vi "Spectrum Recorder.vi"() -> ()   [LabVIEW 2016]
uses:
  Libraries/Spectrum Recorder/Spectrum Recorder Configuration.ctl
  Libraries/Spectrum Recorder/Spectrum Recorder.lvclass
  Libraries/Spectrum Recorder/Spectrum Recorder.lvclass/Spectrum Recorder.ctl
  Libraries/Spectrum Recorder/Write Data file path indicator ref.vi
  Libraries/Spectrum Recorder/Write State ref.vi
  Libraries/Spectrum Recorder/Write Spectrum graph ref.vi
  <vilib>/ErrorRing/Error Ring.xnode
panel:
  in  "Open digitizer":bool
  out "State":bool
  out "Data file path":path=path "C:/Data"
  in  "Exit":bool
  in  "Stop":bool
  in  "Record":bool
  in  "Configuration":T1={"Start"=500000.0, "End"=2000000.0, "Duration"=40.0, "Filter time constant"=0.004, "Repeat (-1: forever)"=1, "Update rate"=1.0, "Data storage folder"=path "C:/Data"} {"Update rate" min=0.001 max=10.0 step=0.001 format="%#_6ps"; "Repeat (-1: forever)" format="%.0p"; "Filter time constant" format="%#_6ps"; "Duration" format="%#_6ps"; "End" format="%#_6pHz"; "Start" format="%#_6pHz"}
  out "Spectrum plot":cluster{dbl[], dbl[]}[](graph)
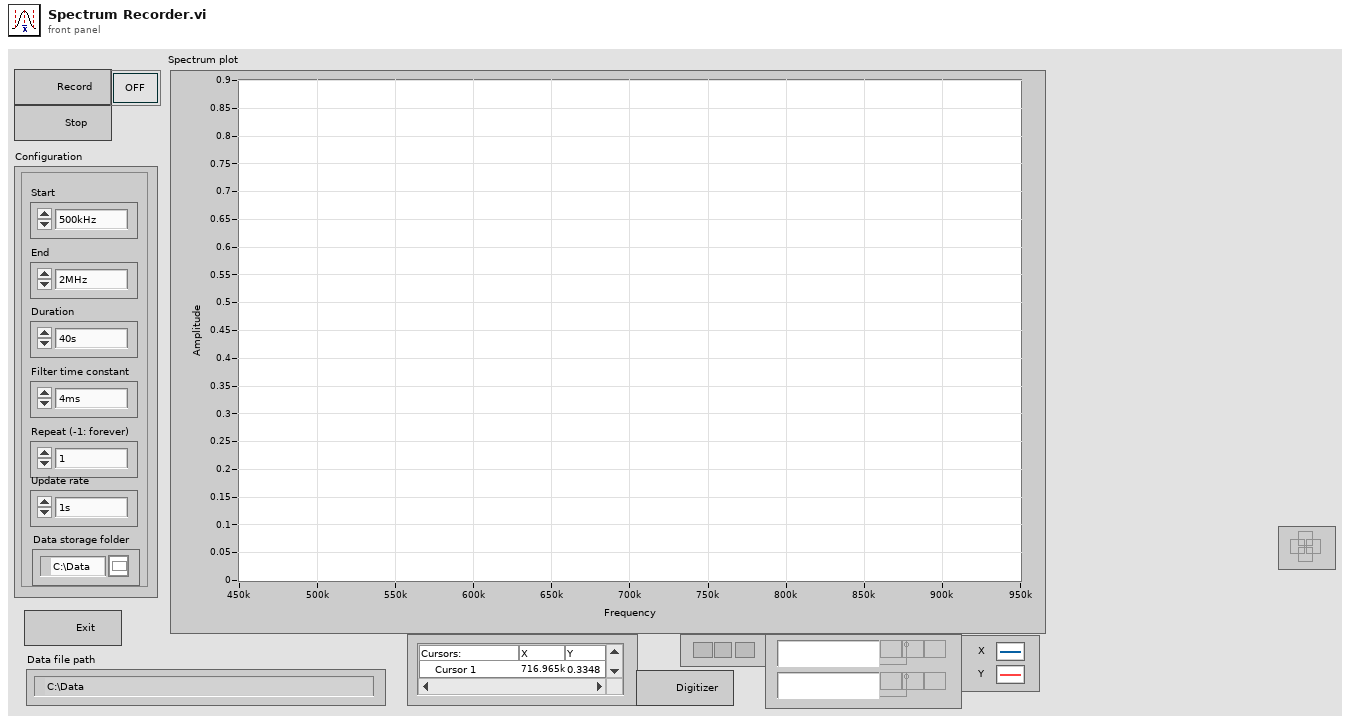
[diagram p1: front panel]
types:
  T1 = typedef "Spectrum Recorder Configuration.ctl" = cluster{"Start":dbl, "End":dbl, "Duration":dbl, "Filter time constant":dbl, "Repeat (-1: forever)":i32, "Update rate":dbl, "Data storage folder":path}
  T2 = enum32{"invalid app kind", "Development System", "Run Time System", "Student Edition", "Embedded LabVIEW", "Evaluation", "Custom"}
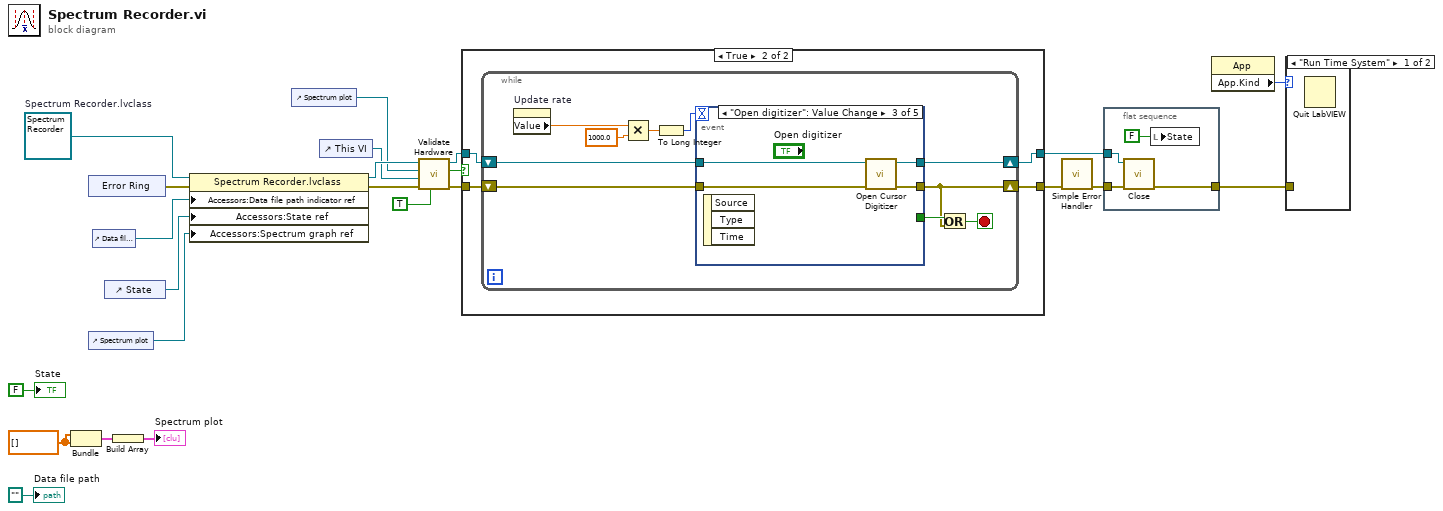
[diagram p0: block diagram]
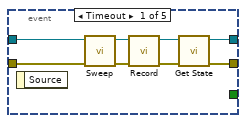
[diagram p4: hidden frame]
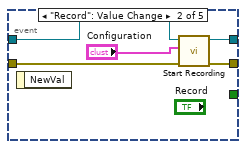
[diagram p5: hidden frame]
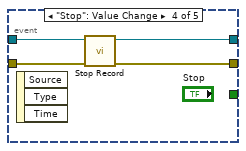
[diagram p6: hidden frame]
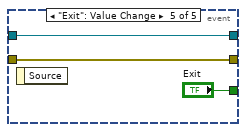
[diagram p7: hidden frame]
diagram:
  w20 = dbl[] []
  w12 = refnum<class "Spectrum Recorder.lvclass"> refnum  # Spectrum Recorder.lvclass
  n1 = Bundle(w20, w20) -> (w19:cluster{dbl[], dbl[]})  [unwired: 1 in]
  n2 = xnode "Error Ring"() -> ("error out"=w23:errorcluster)
  n3 = control-ref of="Spectrum plot"() -> (w17:refnum<vi>)
  n4 = control-ref of="Data file path"() -> (w22:refnum<vi>)
  n5 = control-ref of="State"() -> (w21:refnum<vi>)
  n6 = Build Array(w19) -> (→"Spectrum plot":cluster{dbl[], dbl[]}[])
  n7 = property class="Spectrum Recorder.lvclass"(reference=w12, error in=w23, "Accessors:Data file path indicator ref"=w22, "Accessors:State ref"=w21, "Accessors:Spectrum graph ref"=w17) -> (reference out=w11:refnum<class "Spectrum Recorder.lvclass">, error out=w9:errorcluster)
  n8 = control-ref of="Spectrum plot"() -> (w3:refnum<vi>)
  n9 = control-ref of="This VI"() -> (w1:refnum<vi>)
  n10 = call-dynamic "Validate Hardware.vi"("Interactive"=TRUE, "error in (no error)"=w9, "Pane"=w1, "XY graph ref"=w3, "Spectrum Recorder in"=w11) -> ("error out"=w8:errorcluster, "Valid"=w7:bool, "Spectrum Recorder out"=w10:refnum<class "Spectrum Recorder.lvclass">)  [unwired: 4 in]
  n11 = case shown="True" w7 {
    tunnel: w8 -> [w25 w29]
    tunnel: w10 -> [w24 w28]
    tunnel: [w25 w27] -> w16
    tunnel: [w24 w26] -> w2
    frame False {
    }
    frame True {
      n12 = while {
        shift-right: [w33] -> w26
        shift-left: w28 -> [w34]
        shift-right: [w30] -> w27
        shift-left: w29 -> [w32]
        stop <- w31 stop-if-true
        n13 = property on="Update rate" class="DigNum (strict)"() -> ("Value"=w38:dbl)  [unwired: 2 in, 2 out]
        n14 = Multiply(x=w38, y=1000.0) -> (x*y=w36:dbl)
        n15 = To Long Integer(number=w36) -> (32bit integer=w35:i32)
        n16 = event shown="[2] \"Open digitizer\": Value Change" {
          selector: _ -> [_ _ _ _ _]
          dyn-events: _ -> [_ _ _ _ _]
          timeout: w35 -> [_ _ _ _ _]
          tunnel: [_ _ _ _ "Exit"] -> w39
          tunnel: w34 -> [w45 w50 w54 w59 w62]
          tunnel: [w40 w49 w53 w57 w62] -> w33
          tunnel: w32 -> [w47 w52 w56 w60 w61]
          tunnel: [w42 w51 w55 w58 w61] -> w30
          event Timeout {
            n17 = event-data() -> ()  [unwired: 1 in, 1 out]
            n18 = call-dynamic "Sweep.vi"("error in (no error)"=w47, "Spectrum Recorder in"=w45) -> ("error out"=w46:errorcluster, "Spectrum Recorder out"=w43:refnum<class "Spectrum Recorder.lvclass">)  [unwired: 8 in]
            n19 = call-dynamic "Record.vi"("error in (no error)"=w46, "Spectrum Recorder in"=w43) -> ("error out"=w44:errorcluster, "Spectrum Recorder out"=w41:refnum<class "Spectrum Recorder.lvclass">)  [unwired: 8 in]
            n20 = call-dynamic "Get State.vi"("error in (no error)"=w44, "Spectrum Recorder in"=w41) -> ("error out"=w42:errorcluster, "Spectrum Recorder out"=w40:refnum<class "Spectrum Recorder.lvclass">)  [unwired: 8 in]
          }
          event "Record": Value Change {
            n21 = event-data() -> ()  [unwired: 1 in, 1 out]
            n22 = call-dynamic "Start Recording.vi"("error in (no error)"=w52, "User Configuration"="Configuration", "Spectrum Recorder in"=w50) -> ("error out"=w51:errorcluster, "Spectrum Recorder out"=w49:refnum<class "Spectrum Recorder.lvclass">)  [unwired: 7 in]
          }
          event "Open digitizer": Value Change {
            n23 = event-data() -> ()  [unwired: 1 in, 3 out]
            n24 = call-dynamic "Open Cursor Digitizer.vi"("error in (no error)"=w56, "Spectrum Recorder in"=w54) -> ("error out"=w55:errorcluster, "Spectrum Recorder out"=w53:refnum<class "Spectrum Recorder.lvclass">)  [unwired: 8 in]
          }
          event "Stop": Value Change {
            n25 = event-data() -> ()  [unwired: 1 in, 3 out]
            n26 = call-dynamic "Stop Record.vi"("error in (no error)"=w60, "Spectrum Recorder in"=w59) -> ("error out"=w58:errorcluster, "Spectrum Recorder out"=w57:refnum<class "Spectrum Recorder.lvclass">)  [unwired: 8 in]
          }
          event "Exit": Value Change {
            n27 = event-data() -> ()  [unwired: 1 in, 1 out]
          }
        }
        n28 = Or(x=w39, y=w30) -> (x .or. y?=w31:bool)
      }
    }
  }
  n29 = call <vilib>:"Simple Error Handler.vi"("error in (no error)"=w16) -> ("error out"=w13:errorcluster)  [unwired: 4 in, 4 out]
  n30 = flat-sequence {
    tunnel: w13 -> [w65]
    tunnel: [w64] -> w4
    tunnel: w2 -> [w66]
    frame #0 {
      n31 = call-dynamic "Close.vi"("error in (no error)"=w65, "Spectrum Recorder in"=w66) -> ("error out"=w64:errorcluster)  [unwired: 8 in, 1 out]
      n32 = local write "State"(FALSE ("State")) -> ()
    }
  }
  n33 = property class="App"() -> ("App.Kind"=w5:T2)  [unwired: 2 in, 2 out]
  n34 = case shown="\"Run Time System\"" w5 {
    tunnel: w4 -> [_ _]
    frame "Run Time System" {
      n35 = Quit LabVIEW() -> ()  [unwired: 1 in]
    }
    frame "Development System", Default {
    }
  }
  "Data file path" <- path ""
  "State" <- FALSE ("State")
